vi "multiplierA.vi"(10 "Integration Period (s)":dbl, 11 "Input":T1 {"Input Signal" format="%.2f"; "LOCK-IN Freq" format="%.2f"; "LOCK-IN Phase" format="%.2f"; "Time Constant (sec)" format="%.2f"; "Low-pass filter scope" format="%.2f"; "Time" format="%.2f"; "Spectral Amplitude" format="%.2f"; "Phase Angle" format="%.2f"; "Frequency" format="%.2f"; "Amplitude" format="%.2f"}) -> (1 "ymod":dbl[](array[numeric]), 2 "xmod":dbl[](array[numeric]), 3 "OUTPUT":T2 {"Input Signal" format="%.2f"; "Ch 2 Mult" format="%.2f"; "Ch 1 Mult" format="%.2f"; "LOCK-IN Freq" format="%.2f"; "LOCK-IN Phase" format="%.2f"; "Time Constant (sec)" format="%.2f"; "Low-pass filter slope" format="%.2f"; "Time" format="%.2f"; "Noise Amplitude" format="%.2f"; "Phase Angle" format="%.2f"; "Frequency" format="%.2f"; "Amplitude" format="%.2f"})   [LabVIEW 2023]
doc: "Performs the Lock-In's integration / mixing by multiplying the input signal by the reference signal."
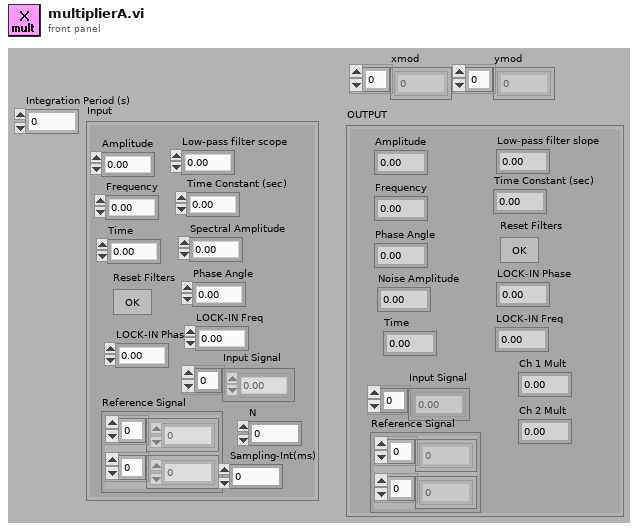
[diagram p1: front panel]
types:
  T1 = cluster{"Amplitude":dbl, "Frequency":dbl, "Phase Angle":dbl, "Spectral Amplitude":dbl, "Time":dbl, "Low-pass filter scope":dbl, "Time Constant (sec)":dbl, "Reset Filters":bool, "LOCK-IN Phase":dbl, "LOCK-IN Freq":dbl, "Sampling-Int(ms)":dbl, "Reference Signal":cluster{dbl[], dbl[]}, "Input Signal":dbl[], "N":i32}
  T2 = cluster{"Amplitude":dbl, "Frequency":dbl, "Phase Angle":dbl, "Noise Amplitude":dbl, "Time":dbl, "Low-pass filter slope":dbl, "Time Constant (sec)":dbl, "Reset Filters":bool, "LOCK-IN Phase":dbl, "LOCK-IN Freq":dbl, "Input Signal":dbl[], "Ch 1 Mult":dbl, "Ch 2 Mult":dbl, "Reference Signal":cluster{dbl[], dbl[]}}
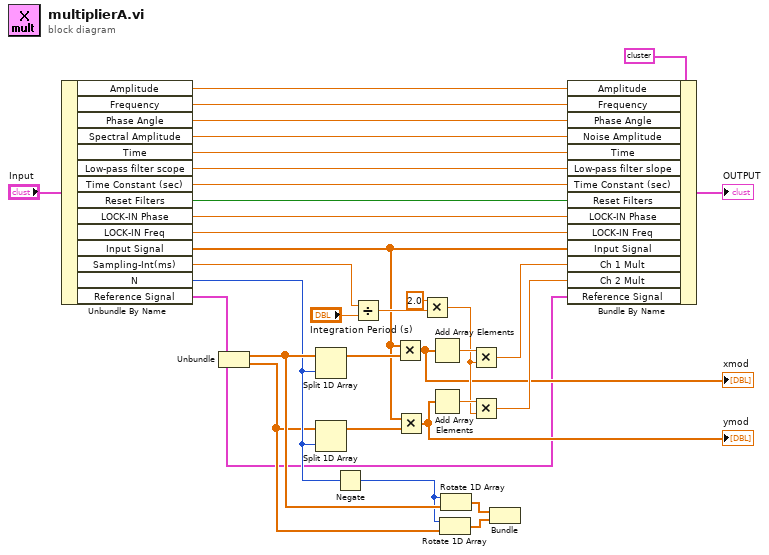
[diagram p0: block diagram]
diagram:
  n1 = Unbundle By Name("Input") -> ("Amplitude"=w34:dbl, "Frequency"=w16:dbl, "Phase Angle"=w33:dbl, "Spectral Amplitude"=w32:dbl, "Time"=w31:dbl, "Low-pass filter scope"=w30:dbl, "Time Constant (sec)"=w29:dbl, "Reset Filters"=w28:bool, "LOCK-IN Phase"=w27:dbl, "LOCK-IN Freq"=w25:dbl, "Input Signal"=w2:dbl[], "Sampling-Int(ms)"=w3:dbl, "N"=w10:i32, "Reference Signal"=w1:cluster{dbl[], dbl[]})
  n2 = Unbundle(w1) -> (w21:dbl[], w7:dbl[])
  n3 = Split 1D Array(array=w21, index=w10) -> (first subarray=w20:dbl[])  [unwired: 1 out]
  n4 = Split 1D Array(array=w7, index=w10) -> (first subarray=w5:dbl[])  [unwired: 1 out]
  n5 = Negate(x=w10) -> (-x=w15:i32)
  n6 = Divide(x=w3, y="Integration Period (s)") -> (x/y=w11:dbl)
  n7 = Multiply(x=w2, y=w20) -> (x*y=w4:dbl[])
  "xmod" <- w4
  n8 = Multiply(x=w2, y=w5) -> (x*y=w9:dbl[])
  "ymod" <- w9
  n9 = Multiply(x=2.0, y=w11) -> (x*y=w12:dbl)
  n10 = Add Array Elements(numeric array=w4) -> (sum=w18:dbl)
  n11 = Add Array Elements(numeric array=w9) -> (sum=w19:dbl)
  n12 = Rotate 1D Array(1:w7, 2:w15) -> (0:w22:dbl[])
  n13 = Rotate 1D Array(1:w21, 2:w15) -> (0:w23:dbl[])
  n14 = Multiply(x=w18, y=w12) -> (x*y=w17:dbl)
  n15 = Multiply(x=w19, y=w12) -> (x*y=w6:dbl)
  n16 = Bundle(w23, w22) -> ()  [unwired: 1 in, 1 out]
  n17 = Bundle By Name(cluster=T2 {"Amplitude"=1.0, "Frequency"=90.0, "Phase Angle"=0.0, "Noise Amplitude"=3.1622776601683794e-12, "Time"=15.5, "Low-pass filter slope"=2.0, "Time Constant (sec)"=3.0, "Reset Filters"=TRUE, "LOCK-IN Phase"=0.0, "LOCK-IN Freq"=90.0, "Input Signal"=[3.6270014704731955e-10, 0.7639707479411351, 0.32806858266099154, 0.03116910771588919, 0.6261334584508225, 0.559016994196243, -0.46661849662936283, -0.683196308630999, -0.06897966261191531, -0.25199859719526513, -0.7694208844477284, -0.1250859172372213, 0.7398902012390709, 0.4067580802859709, 0.007869738850446182, 0.5590169943230116, 0.6364758026279465, -0.3616040548870293, -0.7275301742948549, -0.11980726686689382, -0.1816356320077278, -0.7568653348095259, -0.24672889297442516, 0.697181226573696, 0.48483057948780817, 0.0, 0.48483057963293147, 0.6971812260973207, -0.24672889332109527, -0.7568653348144952, -0.18163563204574137, -0.1198072668350432, -0.7275301744952588, -0.3616040548022246, 0.6364758024591584, 0.5590169943173463, 0.00786973885047025, 0.40675808032800603, 0.7398902013892035, -0.12508591739506292, -0.769420884183334, -0.25199859714365924, -0.06897966261341107, -0.6831963085445812, -0.46661849653327014, 0.5590169940952557, 0.6261334586645678, 0.031169107708940127, 0.32806858266562805, 0.7639707483194247, 3.050194502447735e-10, -0.7639707481316645, -0.3280685826235266, -0.03116910771200357, -0.6261334583012064, -0.5590169945442752, 0.46661849661387955, 0.6831963086207411, 0.06897966261637724, 0.251998597161211, 0.7694208845491353, 0.12508591737979402, -0.7398902015961744, -0.40675808019389864, -0.00786973884866858, -0.5590169943866681, -0.6364758029756332, 0.3616040547369034, 0.7275301742380216, 0.11980726683753752, 0.18163563197239485, 0.7568653349769223, 0.24672889325318684, -0.6971812263598314, -0.4848305795125243, 0.0, -0.4848305794652994, -0.6971812262925658, 0.24672889337578283, 0.7568653350268335, 0.18163563201669025, 0.11980726684926235, 0.727530174431457, 0.36160405447869354, -0.6364758024685663, -0.5590169942792828, -0.007869738852104208, -0.40675808027683447, -0.7398902012745293, 0.1250859170488911, 0.7694208841740288, 0.2519985971529551, 0.0689796626074951, 0.6831963086494821, 0.46661849653975535, -0.5590169941653226, -0.6261334584911336, -0.031169107715581835, -0.32806858260126787, -0.7639707482084847], "Ch 1 Mult"=0.5000000000081768, "Ch 2 Mult"=-1.1719030190704416e-11, "Reference Signal"={array[100000 elements], array[100000 elements]}} ("OUTPUT"), "Amplitude"=w34, "Frequency"=w16, "Phase Angle"=w33, "Noise Amplitude"=w32, "Time"=w31, "Low-pass filter slope"=w30, "Time Constant (sec)"=w29, "Reset Filters"=w28, "LOCK-IN Phase"=w27, "LOCK-IN Freq"=w25, "Input Signal"=w2, "Ch 1 Mult"=w17, "Ch 2 Mult"=w6, "Reference Signal"=w1) -> (→"OUTPUT":T2)
